vi "Load Configuration.vi"(8 "error in (no error)":errorcluster, 11 "Configuration in":refnum<class "Configuration.lvclass">) -> (0 "error out":errorcluster, 2 "Path Loaded From":path, 3 "Configuration out":refnum<class "Configuration.lvclass">)   [LabVIEW 2020, in "Configuration.lvlib" / "Configuration.lvclass"]
uses:
  Configuration.lvclass
  Configuration.lvclass/Configuration.ctl
  <vilib>/Utility/config.llb/NI_LVConfig.lvlib
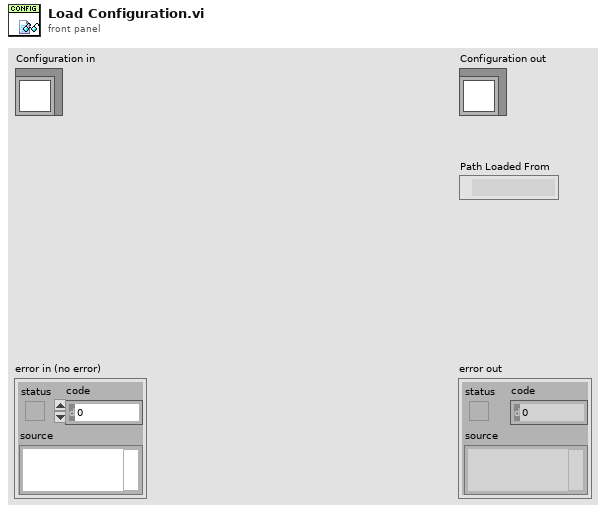
[diagram p1: front panel]
types:
  T1 = typedef "NI_LVConfig.lvlib/Config Data RefNum.ctl" = refnum<k1>
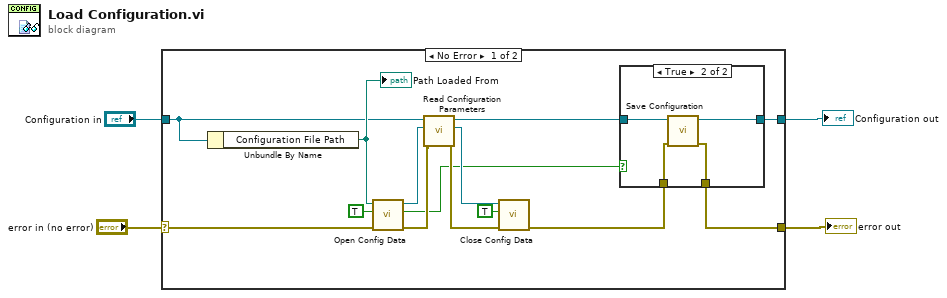
[diagram p0: block diagram]
diagram:
  n1 = case shown="No Error" "error in (no error)" {
    selector: "error in (no error)" -> [w16 w26]
    tunnel: [w6 w26] -> w3
    tunnel: [w8 w25] -> w1
    tunnel: "Configuration in" -> [w14 w25]
    frame No Error {
      n2 = Unbundle By Name(w14) -> ("Configuration File Path"=w18:path)
      "Path Loaded From" <- w18
      n3 = call <vilib>:"Open Config Data.vi"("error in (no error)"=w16, "create file if necessary (T)"=TRUE, "configuration file path"=w18) -> ("error out"=w13:errorcluster, "file created?"=w5:bool, "refnum"=w11:T1)  [unwired: 6 in]
      n4 = call-dynamic "Read Configuration Parameters.vi"("error in (no error)"=w13, "refnum"=w11, "Configuration in"=w14) -> ("error out"=w12:errorcluster, "refnum out"=w10:T1, "Configuration out"=w9:refnum<class "Configuration.lvclass">)  [unwired: 6 in]
      n5 = call <vilib>:"Close Config Data.vi"("error in (no error)"=w12, "write file if changed (T)"=TRUE, "refnum"=w10) -> ("error out"=w7:errorcluster)  [unwired: 7 in, 1 out]
      n6 = case shown="True" w5 {
        tunnel: w9 -> [w20 w24]
        tunnel: [w20 w23] -> w8
        tunnel: w7 -> [w19 w22]
        tunnel: [w19 w21] -> w6
        frame False {
        }
        frame True {
          n7 = call "Save Configuration.vi"("error in (no error)"=w22, "Configuration in"=w24) -> ("error out"=w21:errorcluster, "Configuration out"=w23:refnum<class "Configuration.lvclass">)  [unwired: 7 in, 1 out]
        }
      }
    }
    frame Error {
    }
  }
  "error out" <- w3
  "Configuration out" <- w1
